vi "Name Filter Event.vi"(7 "Label.Text":string, 10 "User Event in":refnum<user-event>) -> (2 "named filter event":cluster{"team filter event":refnum<user-event>})   [LabVIEW 2024]
panel:
  in  "filter event":cluster{"team filter event":refnum<user-event>}
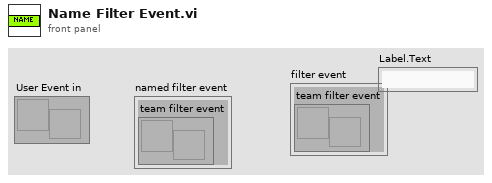
[diagram p1: front panel]
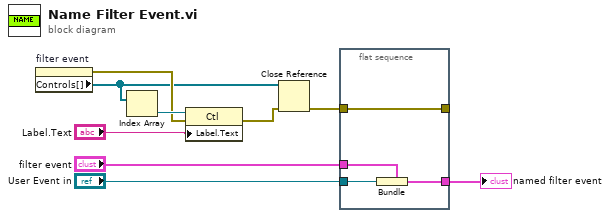
[diagram p0: block diagram]
diagram:
  n1 = property on="filter event" class="Clust (strict)"() -> (error out=w7:errorcluster, "Controls[]"=w6:refnum<vi>[])  [unwired: 2 in, 1 out]
  n2 = Index Array(array=w6) -> (element=w9:refnum<vi>)  [unwired: 1 in]
  n3 = property class="Ctl"(reference=w9, error in=w7, "Label.Text"="Label.Text") -> (error out=w5:errorcluster)  [unwired: 1 out]
  n4 = Close Reference(reference=w6, error in (no error)=w5) -> (error out=w4:errorcluster)
  n5 = flat-sequence {
    tunnel: [w13] -> _
    tunnel: w4 -> [w13]
    tunnel: "User Event in" -> [w12]
    tunnel: "filter event" -> [w11]
    tunnel: [w10] -> w1
    frame #0 {
      n6 = Bundle(cluster=w11, "team filter event"=w12) -> (w10:cluster{"team filter event":refnum<user-event>})
    }
  }
  "named filter event" <- w1
